vi "final_project.vi"() -> ()   [LabVIEW 2019]
panel:
  in  "Path":path
  in  "error in (no error)":errorcluster
  out "error out":errorcluster
  out "String":string
  out "Current row":i32
  out "Array":string[](array[string])
  in  "File A":path
  in  "milliseconds to wait":u32=2000
  out "Row of Value-sets out of range":i32[](array[numeric])
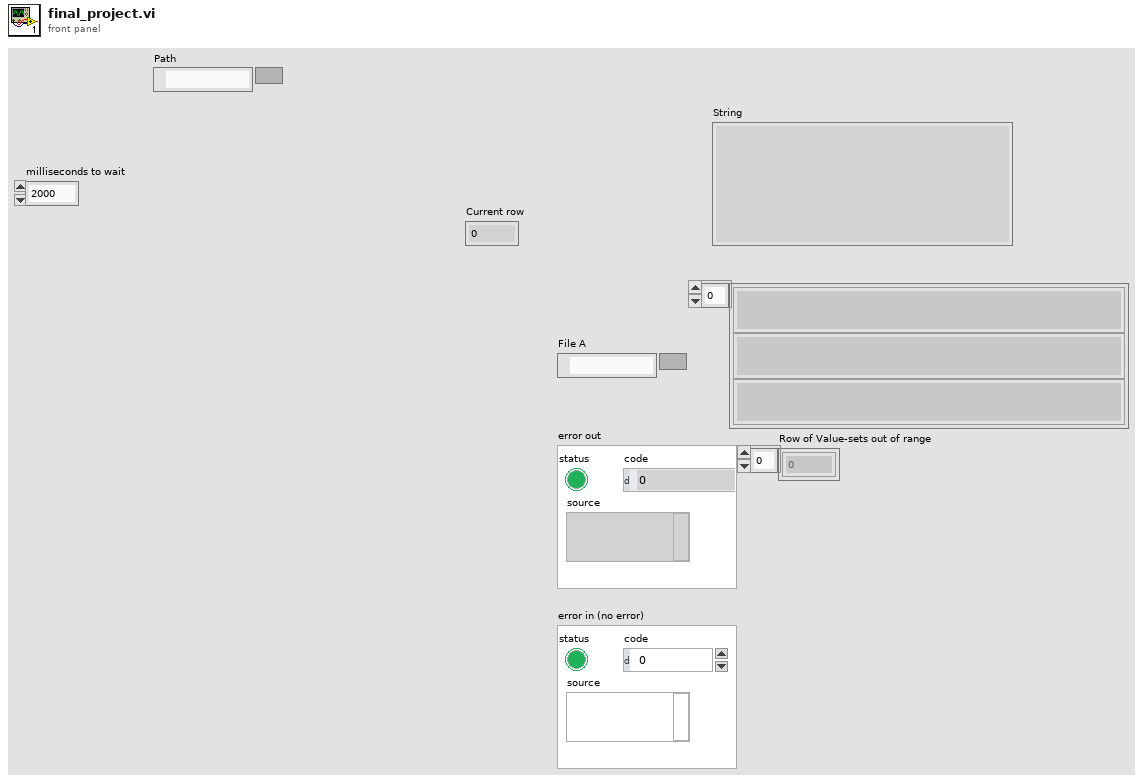
[diagram p1: front panel]
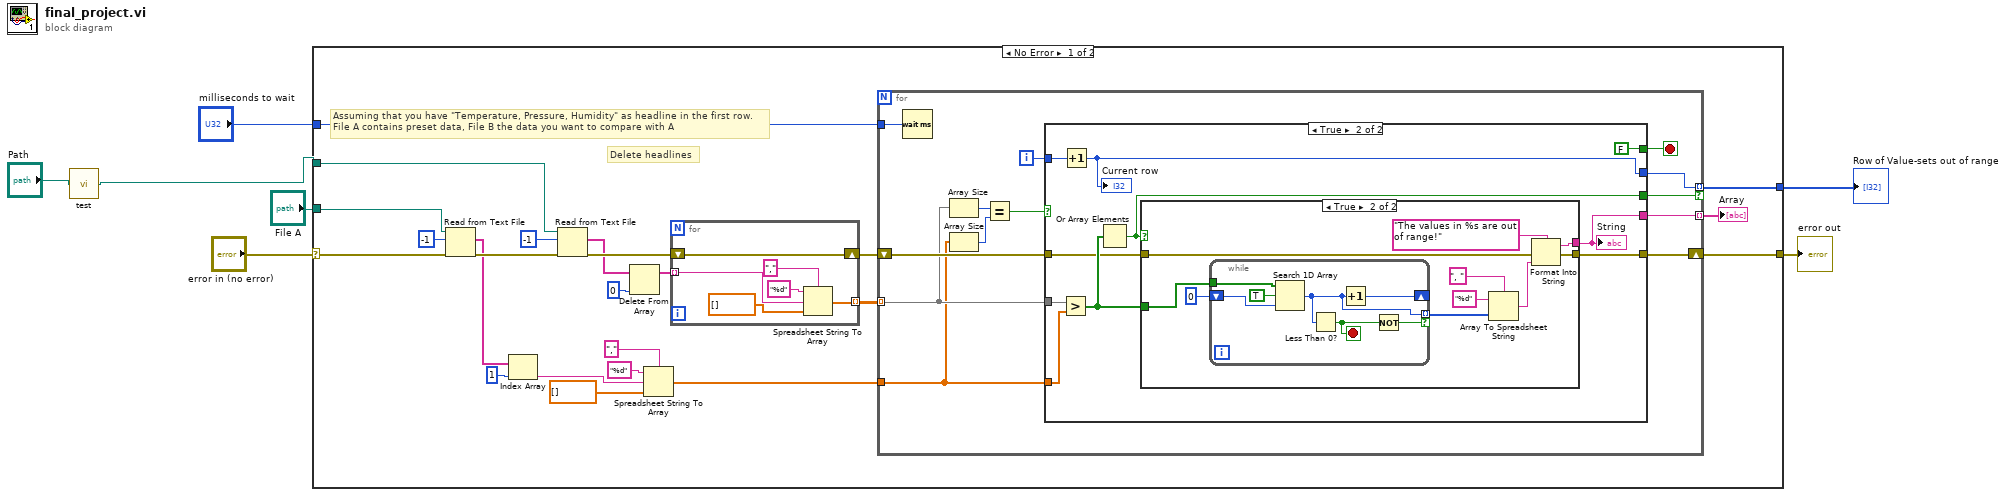
[diagram p0: block diagram]
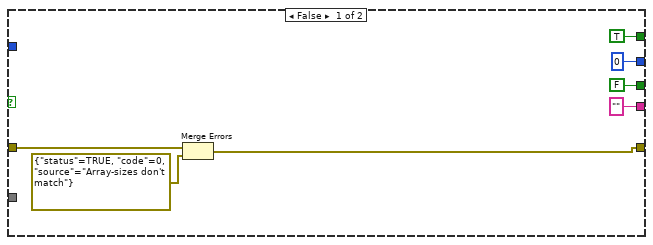
[diagram p2: hidden frame]
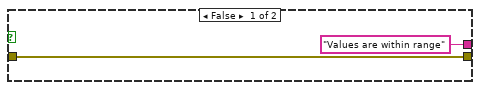
[diagram p3: hidden frame]
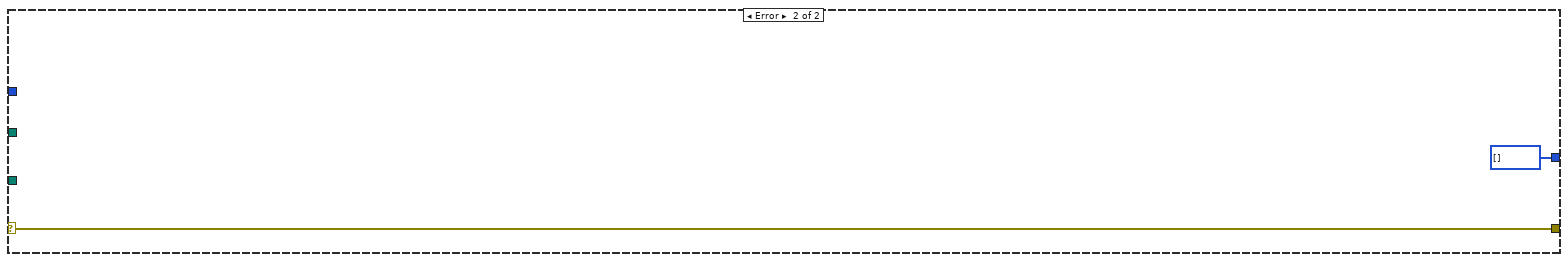
[diagram p4: hidden frame]
diagram:
  n1 = call "test.vi"("Path"="Path") -> ("new file path (Not A Path if cancelled)"=w2:path)
  n2 = case shown="No Error" "error in (no error)" {
    selector: "error in (no error)" -> [w26 w87]
    tunnel: [w13 w87] -> w6
    tunnel: "File A" -> [w30 _]
    tunnel: w2 -> [w29 _]
    tunnel: "milliseconds to wait" -> [w14 _]
    tunnel: [w8 i32[] []] -> w3
    frame No Error {
      # "Delete headlines"
      # "Assuming that you have \"Temperature, Pressure, Humidity\" as headline in the first row.\nFile A contains preset data, File B the data you want to compare with A"
      n3 = Read from Text File(file (use dialog)=w30, count=-1, error in=w26) -> (text=w23:string[], error out=w25:errorcluster)  [unwired: 1 in, 2 out]
      n4 = Index Array(array=w23, index=1) -> (element=w20:string)
      n5 = Read from Text File(file (use dialog)=w29, count=-1, error in=w25) -> (text=w12:string[], error out=w16:errorcluster)  [unwired: 1 in, 2 out]
      n6 = Delete From Array(array=w12, index=0) -> (array with subset deleted=w10:string[])  [unwired: 1 in, 1 out]
      n7 = Spreadsheet String To Array(delimiter (Tab)=",", format string="%d", spreadsheet string=w20, array type (2D Dbl)=dbl[] []) -> (array=w17:dbl[])
      n8 = for {
        tunnel: w10 -> [w82] mode=indexing
        tunnel: [w81] -> w18 mode=indexing
        shift-right: [w80] -> w15
        shift-left: w16 -> [w80]
        n9 = Spreadsheet String To Array(delimiter (Tab)=",", format string="%d", spreadsheet string=w82, array type (2D Dbl)=dbl[] []) -> (array=w81:dbl[])
      }
      n10 = for {
        tunnel: w18 -> [w36] mode=indexing
        tunnel: w17 -> [w35]
        shift-right: [w41] -> w13
        shift-left: w15 -> [w43]
        tunnel: w14 -> [w42]
        tunnel: [w39] -> w9 mode=indexing
        tunnel: [w38] -> w8 mode=indexing if=w37
        i -> [w40]
        stop <- w31 stop-if-true
        n11 = Wait (ms)(milliseconds to wait=w42) -> ()  [unwired: 1 out]
        n12 = Array Size(array=w36) -> (size(s)=w34:i32)
        n13 = Array Size(array=w35) -> (size(s)=w33:i32)
        n14 = Equal?(x=w34, y=w33) -> (x = y?=w32:bool)
        n15 = case shown="True" w32 {
          tunnel: w43 -> [w49 w59]
          tunnel: [w48 w58] -> w41
          tunnel: w40 -> [_ w57]
          tunnel: ["" w56] -> w39
          tunnel: [0 w55] -> w38
          tunnel: [FALSE w54] -> w37
          tunnel: w36 -> [_ w53]
          tunnel: w35 -> [_ w52]
          tunnel: [TRUE FALSE] -> w31
          frame False {
            n16 = Merge Errors(w49, errorcluster {"status"=TRUE, "code"=0, "source"="Array-sizes don't match"} ("error constant")) -> (w48:errorcluster)
          }
          frame True {
            n17 = Greater?(x=w53, y=w52) -> (0:w60:bool[])
            n18 = Increment(x=w57) -> (x+1=w55:i32)
            "Current row" <- w55
            n19 = Or Array Elements(Boolean array=w60) -> (logical OR=w54:bool)
            n20 = case shown="True" w54 {
              tunnel: w60 -> [_ w72]
              tunnel: w59 -> [w62 w66]
              tunnel: [w62 w65] -> w58
              tunnel: ["Values are within range" w63] -> w56
              frame False {
              }
              frame True {
                n21 = while {
                  tunnel: w72 -> [w79]
                  shift-right: [w75] -> _
                  shift-left: 0 -> [w77]
                  tunnel: [w76] -> w70 mode=indexing if=w73
                  stop <- w74 stop-if-true
                  n22 = Search 1D Array(1D array=w79, element=TRUE, start index (0)=w77) -> (index of element=w76:i32)
                  n23 = Less Than 0?(x=w76) -> (x < 0?=w74:bool)
                  n24 = Increment(x=w76) -> (x+1=w75:i32)
                  n25 = Not(x=w74) -> (.not. x?=w73:bool)
                }
                n26 = Array To Spreadsheet String(delimiter (Tab)=", ", array=w70, 3:"%d" ("format string")) -> (spreadsheet string=w67:string)
                n27 = Format Into String(format string="The values in %s are out of range!" ("initial string"), error in=w66, w67) -> (resulting string=w63:string, error out=w65:errorcluster)  [unwired: 1 in]
              }
            }
            "String" <- w56
          }
        }
      }
      "Array" <- w9
    }
    frame Error {
    }
  }
  "error out" <- w6
  "Row of Value-sets out of range" <- w3
